vi "Task Uninit.vi"(8 "error in (no error)":errorcluster, 11 "BasicEventLogger in":refnum<class "BasicEventLogger.lvclass">) -> (0 "error out":errorcluster, 3 "BasicEventLogger out":refnum<class "BasicEventLogger.lvclass">)   [LabVIEW 2020, in "Volatus.lvlib" / "BasicEventLogger.lvclass"]
uses:
  BasicEventLogger.lvclass
  BasicEventLogger.lvclass/BasicEventLogger.ctl
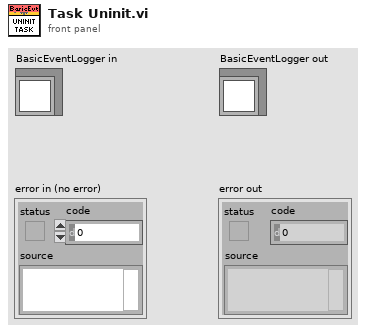
[diagram p1: front panel]
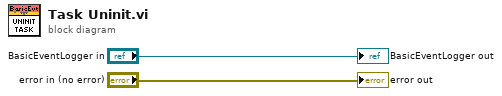
[diagram p0: block diagram]
diagram:
  "error out" <- "error in (no error)"
  "BasicEventLogger out" <- "BasicEventLogger in"
